vi "BuildConnectFlagByte.vi"(8 "error in (no error)":errorcluster, 10 "connFlags":T1) -> (0 "error out":errorcluster, 1 "connFlagByte out":u8)   [LabVIEW 2020, in "BaseMqttMsg.lvclass"]
uses:
  mqttCmd/BaseMqttMsg.lvclass
  mqttTypedef/ConnectionFlags.ctl
  mqttTypedef/QosLevel.ctl
  MQTT Client.lvclass
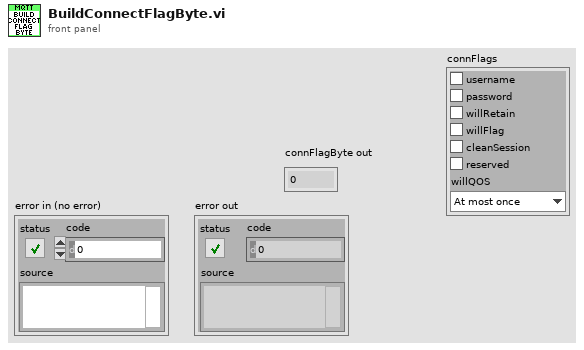
[diagram p1: front panel]
types:
  T1 = typedef "MQTT Client.lvclass/ConnectionFlags.ctl" = cluster{"user name":bool, "password":bool, "will retain":bool, "will flag":bool, "clean session":bool, "reserved":bool, "willQOS":T2}
  T2 = typedef "BaseMqttMsg.lvclass/QosLevel.ctl" = enum8{"At most once", "At least once", "Exactly once", "Reserved"}
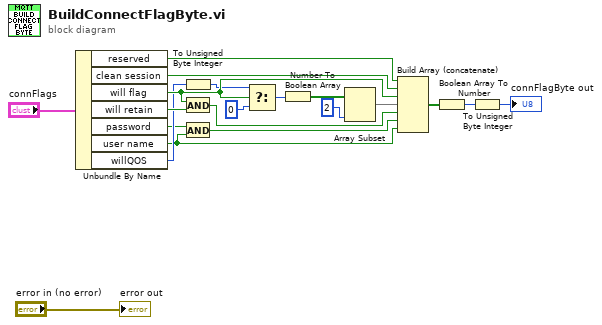
[diagram p0: block diagram]
diagram:
  n1 = Unbundle By Name("connFlags") -> ("reserved"=w18:bool, "clean session"=w19:bool, "will flag"=w9:bool, "will retain"=w11:bool, "password"=w4:bool, "user name"=w3:bool, "willQOS"=w8:T2)
  n2 = To Unsigned Byte Integer(number=w8) -> (unsigned 8bit integer=w7:u8)
  n3 = And(x=w9, y=w11) -> (x .and. y?=w10:bool)
  n4 = And(x=w4, y=w3) -> (x .and. y?=w2:bool)
  n5 = Select(t=w7, s=w9, f=u8 0) -> (s? t:f=w6:u8)
  n6 = Number To Boolean Array(number=w6) -> (Boolean array=w17:bool[])
  n7 = Array Subset(array=w17, length=2) -> (w15:bool[])  [unwired: 1 in]
  n8 = Build Array (concatenate)(w18, w19, w9, w15, w10, w2, w3) -> (w14:bool[])
  n9 = Boolean Array To Number(Boolean array=w14) -> (number=w13:u32)
  n10 = To Unsigned Byte Integer(number=w13) -> (unsigned 8bit integer=→"connFlagByte out":u8)
  "error out" <- "error in (no error)"
